vi "insertion sort.vi"(11 "Array in":dbl[](array[numeric])) -> (2 "Waveform Graph":dbl[](graph), 3 "Array out":dbl[](array[numeric]))   [LabVIEW 2014]
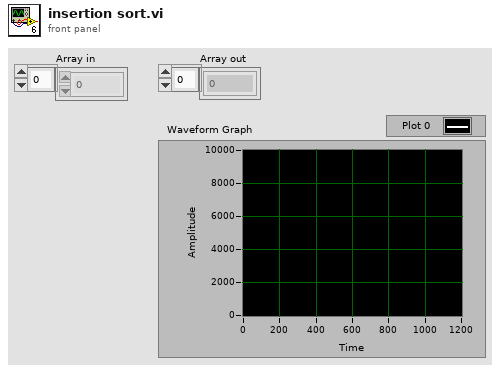
[diagram p1: front panel]
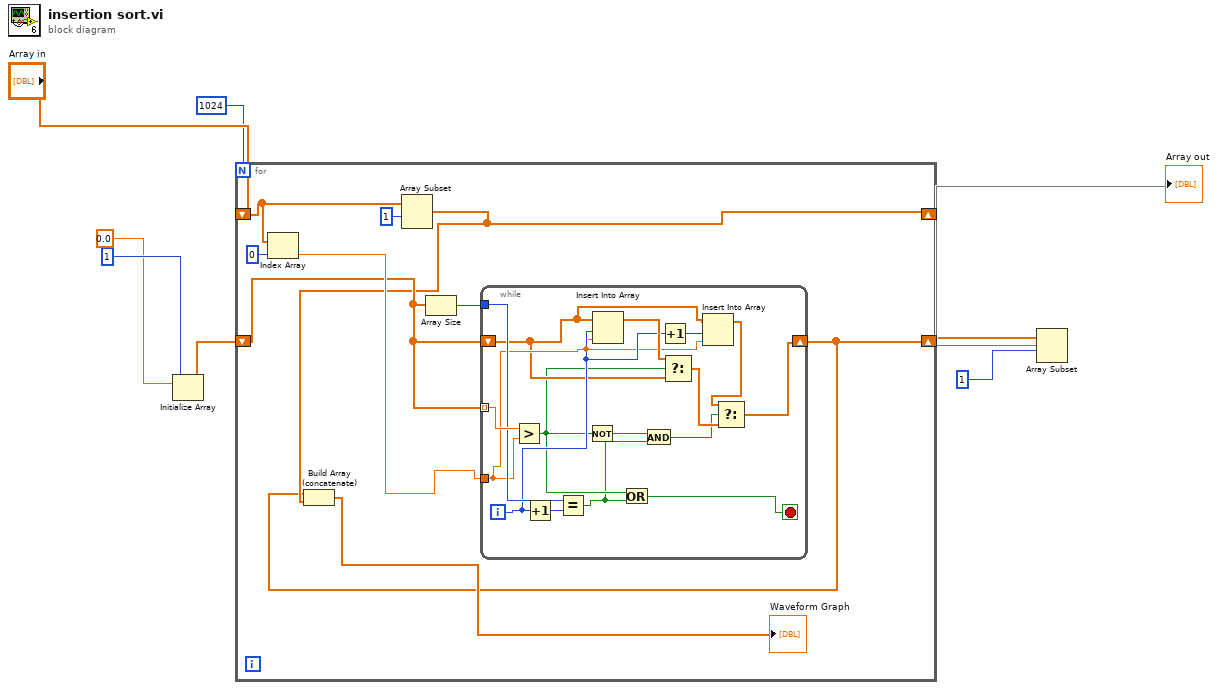
[diagram p0: block diagram]
diagram:
  n1 = Initialize Array(0.0 ("element"), 1 ("dimension size")) -> (w4:dbl[])
  n2 = for {
    N: 1024 -> [_]
    shift-right: [w9] -> w1
    shift-left: w4 -> [w13]
    shift-right: [w10] -> _
    shift-left: "Array in" -> [w12]
    n3 = Index Array(array=w12, index=0) -> (element=w16:dbl)
    n4 = Array Subset(array=w12, index=1) -> (w10:dbl[])  [unwired: 1 in]
    n5 = Array Size(array=w13) -> (size(s)=w17:i32)
    n6 = while {
      tunnel: w13 -> [w33] mode=indexing
      tunnel: w17 -> [w32]
      shift-right: [w22] -> w9
      shift-left: w13 -> [w24]
      tunnel: w16 -> [w26]
      i -> [w28]
      stop <- w30 stop-if-true
      n7 = Greater?(x=w33, y=w26) -> (0:w21:bool)
      n8 = Increment(x=w28) -> (x+1=w31:i32)
      n9 = Equal?(x=w32, y=w31) -> (x = y?=w20:bool)
      n10 = Not(x=w21) -> (.not. x?=w19:bool)
      n11 = Insert Into Array(array=w24, index=w28, new element=w26) -> (w29:dbl[])
      n12 = Or(x=w21, y=w20) -> (x .or. y?=w30:bool)
      n13 = And(x=w19, y=w20) -> (x .and. y?=w18:bool)
      n14 = Increment(x=w28) -> (x+1=w27:i32)
      n15 = Select(t=w29, s=w21, f=w24) -> (s? t:f=w23:dbl[])
      n16 = Insert Into Array(array=w24, index=w27, new element=w26) -> (w25:dbl[])
      n17 = Select(t=w25, s=w18, f=w23) -> (s? t:f=w22:dbl[])
    }
    n18 = Build Array (concatenate)(w9, w10) -> (→"Waveform Graph":dbl[])
  }
  n19 = Array Subset(array=w1, index=1) -> (→"Array out":dbl[])  [unwired: 1 in]
